vi "RSZVB Set Pulse Generator Mode.vi"(8 "error in (no error)":errorcluster {"code" format="%.0x"}, 9 "Pulse Mode (0)":i32(ring) items=["Channel Specific", "Continuous Pulse"], 10 "Channel (1)":i32=1, 11 "VISA session":refnum<visa-resource-name>) -> (0 "error out":errorcluster {"code" format="%.0x"}, 3 "dup VISA session":refnum<visa-resource-name>)   [LabVIEW 2011]
doc: "This VI selects the channel-specific or continuous pulse mode.\n\nNote(s):\n\n(1) This VI is available only with option R&S ZVA-K27.\n\nRemote-control command(s):\n[SENSe<Ch>:]PULSe:GENerator<gen_no>:MODE CSPecific | CONTinuous"
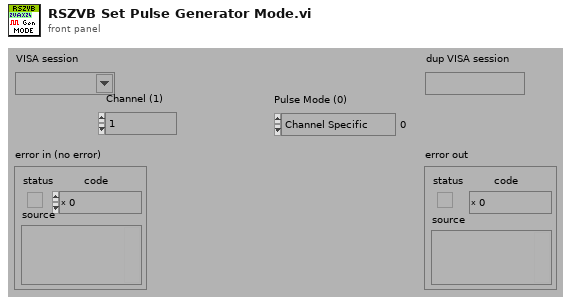
[diagram p1: front panel]
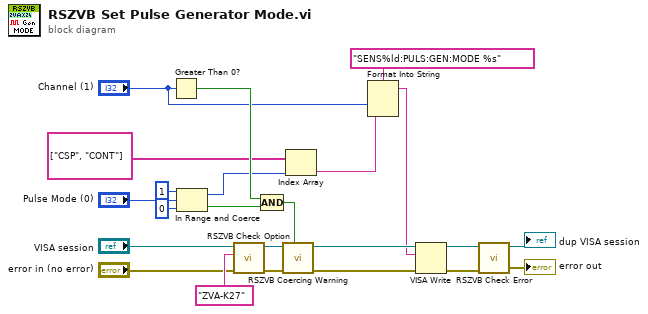
[diagram p0: block diagram]
diagram:
  n1 = Greater Than 0?(x="Channel (1)") -> (x > 0?=w10:bool)
  n2 = In Range and Coerce(upper limit=1, x="Pulse Mode (0)", lower limit=0) -> (coerced(x)=w9:i32, In Range?=w11:bool)
  n3 = call "RSZVB Check Option.vi"("error in (no error)"="error in (no error)", "Options"="ZVA-K27", "VISA session"="VISA session") -> ("error out"=w17:errorcluster, "dup VISA session"=w16:refnum<visa-resource-name>)  [unwired: 7 in]
  n4 = Compound Arithmetic op=AND(w10, w11) -> (w13:bool)
  n5 = call "RSZVB Coercing Warning.vi"("In Range?"=w13, "error in (no error)"=w17, "VISA session"=w16) -> ("error out"=w22:errorcluster, "dup VISA session"=w23:refnum<visa-resource-name>)  [unwired: 7 in]
  n6 = Index Array(array=string[] ["CSP", "CONT"], index=w9) -> (element=w3:string)
  n7 = Format Into String(format string="SENS%ld:PULS:GEN:MODE %s", "Channel (1)", w3) -> (resulting string=w19:string)  [unwired: 2 in, 1 out]
  n8 = VISA Write(VISA resource name=w23, write buffer=w19, error in (no error)=w22) -> (VISA resource name out=w20:refnum<visa-resource-name>, error out=w21:errorcluster)  [unwired: 1 out]
  n9 = call "RSZVB Check Error.vi"("error in (no error)"=w21, "VISA session"=w20) -> ("error out"=→"error out":errorcluster, "dup VISA session"=→"dup VISA session":refnum<visa-resource-name>)  [unwired: 8 in]
